vi "Set Bind Port.vi"(8 "error in (no error)":errorcluster, 10 "Bind Port":u16, 11 "Server Config in":refnum<class "Server Config.lvclass">) -> (0 "error out":errorcluster, 3 "Server Config out":refnum<class "Server Config.lvclass">)   [LabVIEW 2020, in "Examples.lvlib" / "Server Config.lvclass"]
uses:
  Server Config.lvclass
  Server Config.lvclass/Server Config.ctl
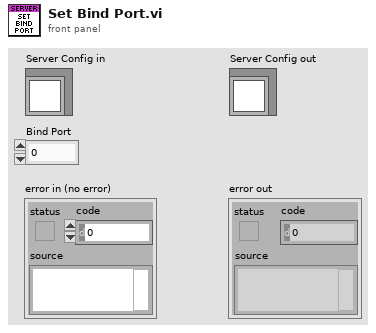
[diagram p1: front panel]
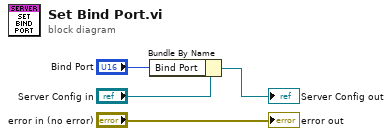
[diagram p0: block diagram]
diagram:
  n1 = Bundle By Name(cluster="Server Config in", "Bind Port"="Bind Port") -> (→"Server Config out":refnum<class "Server Config.lvclass">)
  "error out" <- "error in (no error)"
